vi "Read Denuder Bypass.vi"(8 "error in (no error)":errorcluster, 11 "ePAS in":refnum<class "ePAS.lvclass">) -> (0 "error out":errorcluster, 2 "Denuder Bypass":refnum<k21>="PAS_TEC_AO", 3 "ePAS out":refnum<class "ePAS.lvclass">)   [LabVIEW 2014, in "ePAS Library.lvlib" / "ePAS.lvclass"]
uses:
  ePAS.lvclass
  ePAS.lvclass/ePAS.ctl
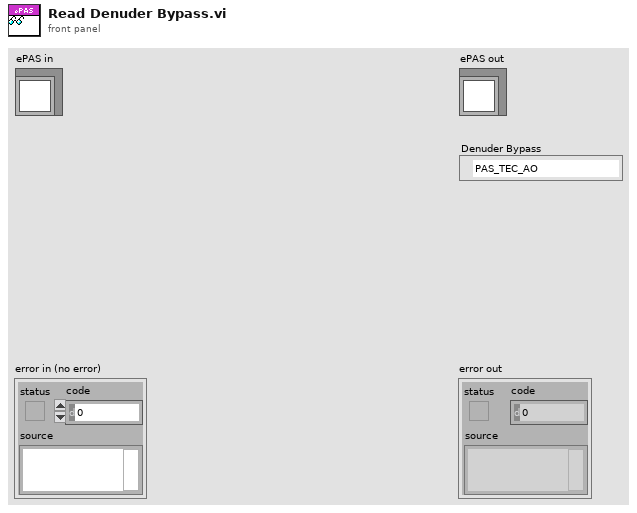
[diagram p1: front panel]
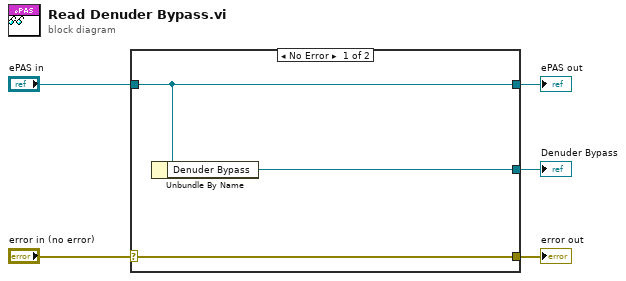
[diagram p0: block diagram]
diagram:
  n1 = case shown="No Error" "error in (no error)" {
    selector: "error in (no error)" -> [w8 w9]
    tunnel: [w8 w9] -> w4
    tunnel: [w7 w10] -> w2
    tunnel: "ePAS in" -> [w7 w10]
    tunnel: [w6 _] -> w1
    frame No Error {
      n2 = Unbundle By Name(w7) -> ("Denuder Bypass"=w6:refnum<k21>)
    }
    frame Error {
    }
  }
  "error out" <- w4
  "ePAS out" <- w2
  "Denuder Bypass" <- w1
